vi "Send Aliases to Notebook.vi"(8 "Satistics Aliases":i32[](array[numeric]), 9 "Descriptions Array":string[](array[string]), 10 "Definitions Array":string[](array[string]), 11 "Aliases Array":string[](array[string])) -> ()   [LabVIEW 2021, in "Formula.lvlib"]
uses:
  Formula.lvlib
  Notebook/Notebook.lvlib
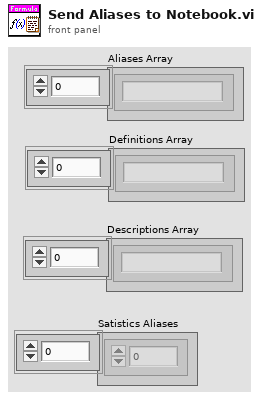
[diagram p1: front panel]
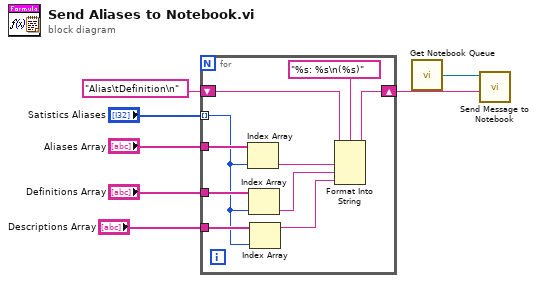
[diagram p0: block diagram]
diagram:
  n1 = for {
    tunnel: "Satistics Aliases" -> [w9] mode=indexing
    tunnel: "Aliases Array" -> [w17]
    tunnel: "Definitions Array" -> [w16]
    shift-right: [w13] -> w3
    shift-left: "Alias\tDefinition\n" ("format string") -> [w15]
    tunnel: "Descriptions Array" -> [w10]
    n2 = Index Array(array=w17, index=w9) -> (element=w12:string)
    n3 = Index Array(array=w16, index=w9) -> (element=w11:string)
    n4 = Index Array(array=w10, index=w9) -> (element=w8:string)
    n5 = Format Into String(format string="%s: %s\n(%s)", initial string=w15, w12, w11, w8) -> (resulting string=w13:string)  [unwired: 1 in, 1 out]
  }
  n6 = call "Get Notebook Queue.vi"() -> ("Notebook Queue"=w1:refnum<queue>)  [unwired: 9 in]
  n7 = call "Send Message to Notebook.vi"("Message"=w3, "Notebook Queue"=w1) -> ()  [unwired: 6 in, 2 out]
